vi "Rename.vi"(8 "error in (no error)":errorcluster, 9 "New name":string, 10 "ProjectItem Refnum":refnum<vi>, 11 "PPL in":refnum<class "NI_AB_API_PPL.lvclass">) -> (0 "error out":errorcluster, 3 "PPL out":refnum<class "NI_AB_API_PPL.lvclass">)   [LabVIEW 2020, in "NI_AB_API_PPL.lvclass"]
uses:
  <vilib>/AppBuilder/AB_API/PPL/NI_AB_API_PPL.lvclass
  e:/builds/penguin/labview/branches/2020/dev/dist/vi.lib/AppBuilder/AB_API/Build/NI_AB_API_Build.lvclass
  <vilib>/AppBuilder/AB_Classes/PackedLib/AB_PackedLibrary.lvclass
  e:/builds/penguin/labview/branches/2020/dev/dist/vi.lib/AppBuilder/AB_Classes/Build/AB_Build.lvclass
  <vilib>/AppBuilder/AB_Source_Inclusion.ctl
  <vilib>/AppBuilder/AB_Classes/Build/AB_Build.lvclass
  <vilib>/AppBuilder/AB_API/Build/NI_AB_API_Build.lvclass
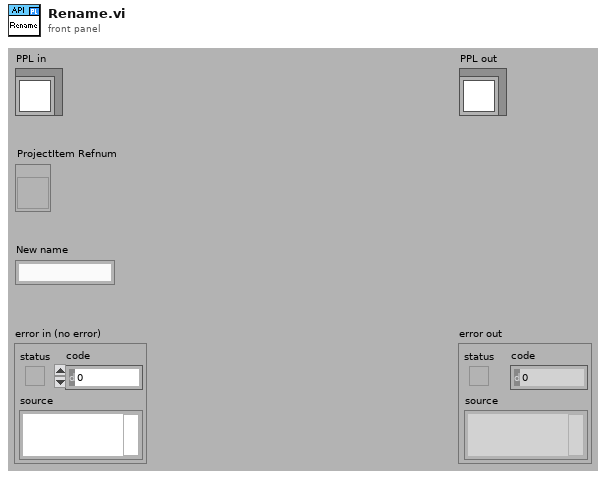
[diagram p1: front panel]
types:
  T1 = typedef "AB_Source_Inclusion.ctl" = enum16{"IncludeIfReferenced", "Include", "Exclude", "TopLevel"}
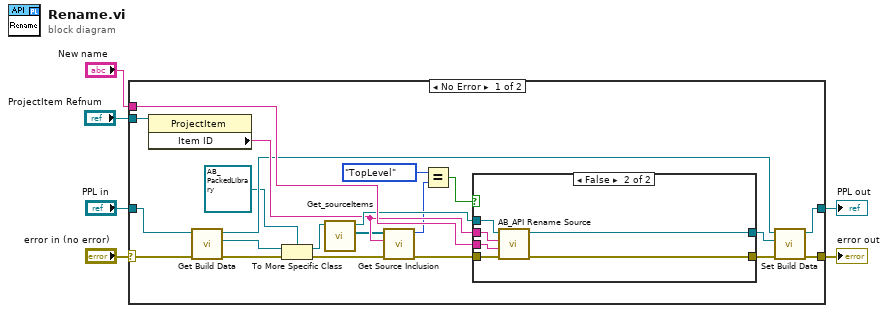
[diagram p0: block diagram]
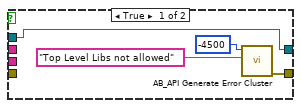
[diagram p2: hidden frame]
diagram:
  n1 = case shown="No Error" "error in (no error)" {
    selector: "error in (no error)" -> [w12 w39]
    tunnel: [w18 w39] -> w5
    tunnel: [w16 w38] -> w3
    tunnel: "PPL in" -> [w14 w38]
    tunnel: "New name" -> [w27 _]
    tunnel: "ProjectItem Refnum" -> [w26 _]
    frame No Error {
      n2 = property class="ProjectItem"(reference=w26) -> ("Item ID"=w24:string)  [unwired: 1 in, 2 out]
      n3 = call <vilib>:"Get Build Data.vi"("error in (no error)"=w12, "NI_AB_API_Build in"=w14) -> ("error out"=w11:errorcluster, "AB_Build.lvclass"=w8:refnum<class "AB_Build.lvclass">, "NI_AB_API_Build out"=w13:refnum<class "NI_AB_API_PPL.lvclass">)  [unwired: 7 in]
      n4 = To More Specific Class(target class=refnum<class "AB_PackedLibrary.lvclass"> refnum ("AB_PackedLibrary.lvclass"), reference=w8, error in=w11) -> (specific class reference=w7:refnum<class "AB_PackedLibrary.lvclass">, error out=w10:errorcluster)
      n5 = call <vilib>:"Get_sourceItems.vi"("Class in"=w7) -> ("sourceItems"=w23:refnum<class "AB_Source.lvclass">[], "Class out"=w25:refnum<class "AB_PackedLibrary.lvclass">)  [unwired: 8 in, 1 out]
      n6 = call <vilib>:"Get Source Inclusion.vi"("error IO"=w10, "Item ID"=w24, "sourceItems"=w23) -> ("error out"=w22:errorcluster, "sourceInclusion"=w19:T1)  [unwired: 7 in]
      n7 = Equal?(x=AB_Source_Inclusion."TopLevel", y=w19) -> (x = y?=w21:bool)
      n8 = case shown="False" w21 {
        tunnel: w27 -> [_ w37]
        tunnel: [w28 w36] -> w17
        tunnel: [w31 w35] -> w15
        tunnel: w25 -> [w31 w34]
        tunnel: w24 -> [_ w33]
        tunnel: w22 -> [_ w32]
        frame True {
          n9 = call <vilib>:"AB_API Generate Error Cluster.vi"("Additional Message"="Top Level Libs not allowed", "Code"=-4500) -> ("error out"=w28:errorcluster)  [unwired: 9 in]
        }
        frame False {
          n10 = call <vilib>:"AB_API Rename Source.vi"("error in (no error)"=w32, "New name"=w37, "source item ID"=w33, "Build in"=w34) -> ("error out"=w36:errorcluster, "Build out"=w35:refnum<class "AB_PackedLibrary.lvclass">)  [unwired: 6 in]
        }
      }
      n11 = call <vilib>:"Set Build Data.vi"("error in (no error)"=w17, "AB_Build.lvclass"=w15, "NI_AB_API_Build in"=w13) -> ("error out"=w18:errorcluster, "NI_AB_API_Build out"=w16:refnum<class "NI_AB_API_PPL.lvclass">)  [unwired: 7 in]
    }
    frame Error {
    }
  }
  "error out" <- w5
  "PPL out" <- w3
